vi "calcANDmoveSD.vi"(1 "timedelays":dbl[](array[numeric]), 2 "Value":i32, 3 "Cluster in":T1, 4 "DelaysTab":enum32{"Mode Normale", "Table"}(ring)) -> (0 "Real delay time, ps":dbl)   [LabVIEW 2015]
uses:
  controls/clustercontrols-measerument.ctl
  Classes/Experiment.lvclass
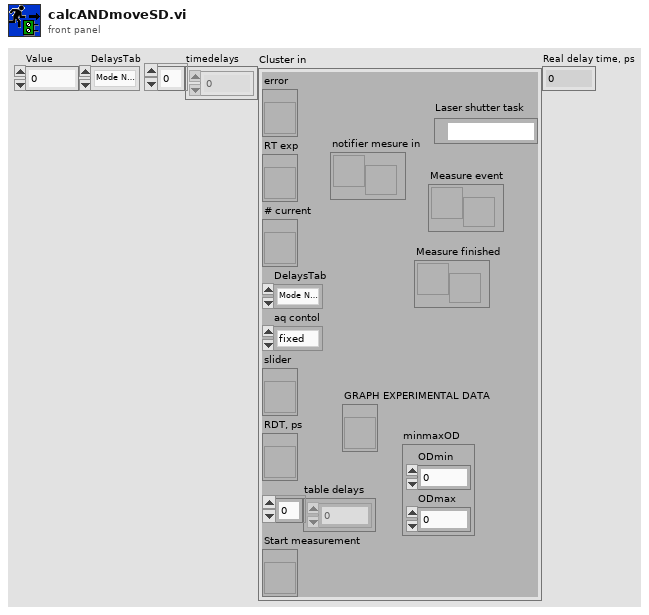
[diagram p1: front panel]
types:
  T1 = typedef "clustercontrols-measerument.ctl" = cluster{"error":refnum<vi>, "RT exp":refnum<vi>, "# current":refnum<vi>, "Start measurement":refnum<vi>, "GRAPH EXPERIMENTAL DATA":refnum<vi>, "DelaysTab":enum32{"Mode Normale", "Table"}, "slider":refnum<vi>, "aq contol":enum32{"fixed", "automatic", "fixed-auto"}, "RDT, ps":refnum<vi>, "table delays":dbl[], "notifier mesure in":refnum<notifier>, "Measure finished":refnum<user-event>, "Measure event":refnum<user-event>, "Laser shutter task":refnum<k21>, "minmaxOD":cluster{"ODmin":dbl, "ODmax":dbl}}
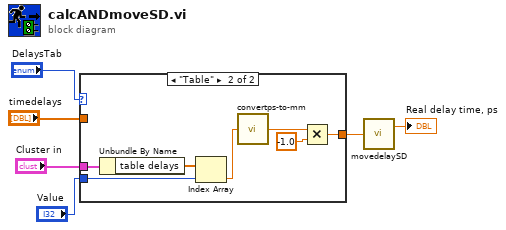
[diagram p0: block diagram]
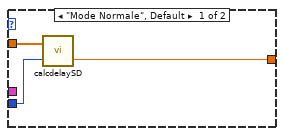
[diagram p2: hidden frame]
diagram:
  n1 = case shown="\"Table\"" "DelaysTab" {
    tunnel: "Value" -> [w9 w16]
    tunnel: [w8 w12] -> w3
    tunnel: "timedelays" -> [w7 _]
    tunnel: "Cluster in" -> [_ w10]
    frame "Mode Normale", Default {
      n2 = call "calcdelaySD.vi"("current point"=w9, "timedelays"=w7) -> ("Delay, mm"=w8:dbl)  [unwired: 1 in]
    }
    frame "Table" {
      n3 = Unbundle By Name(w10) -> ("table delays"=w11:dbl[])
      n4 = Index Array(array=w11, index=w16) -> (element=w13:dbl)
      n5 = call "convertps-to-mm.vi"("ps"=w13) -> ("mm"=w14:dbl)
      n6 = Multiply(x=w14, y=-1.0) -> (x*y=w12:dbl)
    }
  }
  n7 = call "movedelaySD.vi"("Delay, mm"=w3) -> ("Real delay time, ps"=→"Real delay time, ps":dbl)  [unwired: 1 out]
